vi "_TreeItem.Property.Get.Dictionary.vi"(8 "error in (no error)":errorcluster, 11 "DictionaryProperty":refnum<k39>) -> (0 "error out":errorcluster, 2 "Dictionary Variant":variant, 3 "DictionaryProperty out":refnum<k39>)   [LabVIEW 2027, in "Advanced System Definition.lvlib"]
uses:
  SysDef API/Advanced System Definition.lvlib
  C:/NetCoreDLL/NationalInstruments.VeriStand.SystemStorage.dll
  NetCoreDLL/NationalInstruments.VeriStand.SystemStorage.dll
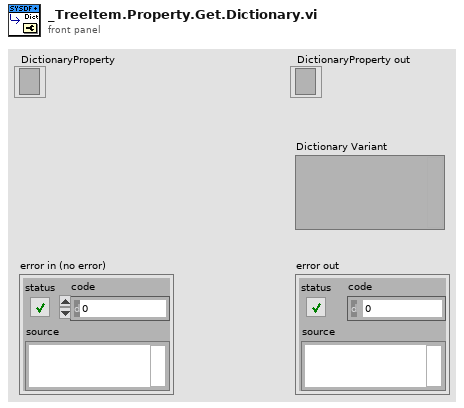
[diagram p1: front panel]
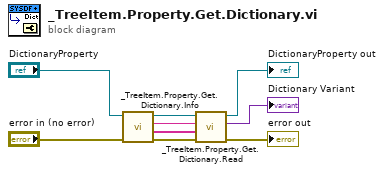
[diagram p0: block diagram]
diagram:
  n1 = call "_TreeItem.Property.Get.Dictionary.Info.vi"("error in (no error)"="error in (no error)", "NationalInstruments.VeriStand.SystemStorage.DictionaryProperty"="DictionaryProperty") -> ("error out"=w7:errorcluster, "Keys"=w4:string[], "DictionaryType"=w5:string, "NationalInstruments.VeriStand.SystemStorage.DictionaryProperty"=w6:refnum<k39>)  [unwired: 6 in]
  n2 = call "_TreeItem.Property.Get.Dictionary.Read.vi"("error in (no error)"=w7, "Keys"=w4, "Type"=w5, "NationalInstruments.VeriStand.SystemStorage.DictionaryProperty"=w6) -> ("error out"=→"error out":errorcluster, "Dictionary Variant"=→"Dictionary Variant":variant, "NationalInstruments.VeriStand.SystemStorage.DictionaryProperty"=→"DictionaryProperty out":refnum<k39>)  [unwired: 5 in]
